vi "Close File.vi"(8 "error in (no error)":errorcluster, 11 "Logger in":refnum<class "Logger.lvclass">) -> (0 "error out":errorcluster, 1 "Actually closed":bool, 2 "File Path":path, 3 "Logger out":refnum<class "Logger.lvclass">)   [LabVIEW 2016, in "Logger.lvclass"]
uses:
  Logger.lvclass
  Logger.lvclass/Logger.ctl
  Read File.lvclass.vi
  Write File.lvclass.vi
  NHMFL_Core/Libraries/File/File Class/File.lvclass
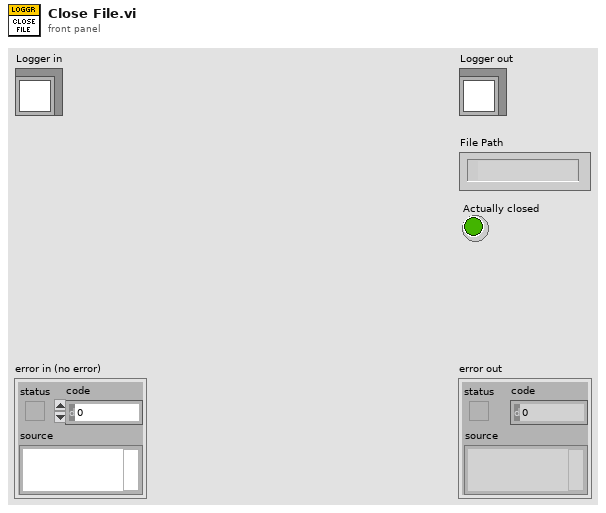
[diagram p1: front panel]
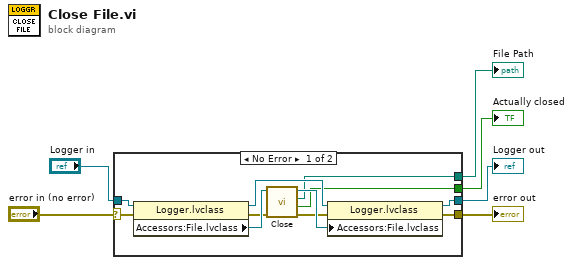
[diagram p0: block diagram]
diagram:
  n1 = case shown="No Error" "error in (no error)" {
    selector: "error in (no error)" -> [w17 w19]
    tunnel: [w15 w19] -> w5
    tunnel: [w13 w18] -> w3
    tunnel: "Logger in" -> [w16 w18]
    tunnel: [w8 _] -> w2
    tunnel: [w7 _] -> w1
    frame No Error {
      n2 = property class="Logger.lvclass"(reference=w16, error in=w17) -> (reference out=w14:refnum<class "Logger.lvclass">, error out=w10:errorcluster, "Accessors:File.lvclass"=w12:refnum<class "File.lvclass">)
      n3 = call-dynamic "Close.vi"("error in (no error)"=w10, "File in"=w12) -> ("error out"=w9:errorcluster, "Actually closed"=w8:bool, "File Path"=w7:path, "File out"=w11:refnum<class "File.lvclass">)  [unwired: 6 in]
      n4 = property class="Logger.lvclass"(reference=w14, error in=w9, "Accessors:File.lvclass"=w11) -> (reference out=w13:refnum<class "Logger.lvclass">, error out=w15:errorcluster)
    }
    frame Error {
    }
  }
  "error out" <- w5
  "Logger out" <- w3
  "Actually closed" <- w2
  "File Path" <- w1
